vi "Wertaenderung Systemeinstellungen.vi"(11 "error in (no error)":errorcluster caption="Fehler (Eingang, kein Fehler)", 13 "Aktion":T1) -> (4 "Tests":T2, 15 "error out":errorcluster caption="Fehler (Ausgang)")   [LabVIEW 2020, in "EPA 1065.lvlib"]
uses:
  EPA 1065.lvlib
  Aktive Tests Cluster.ctl
  Aktion Wertaenderung Gasliste.ctl
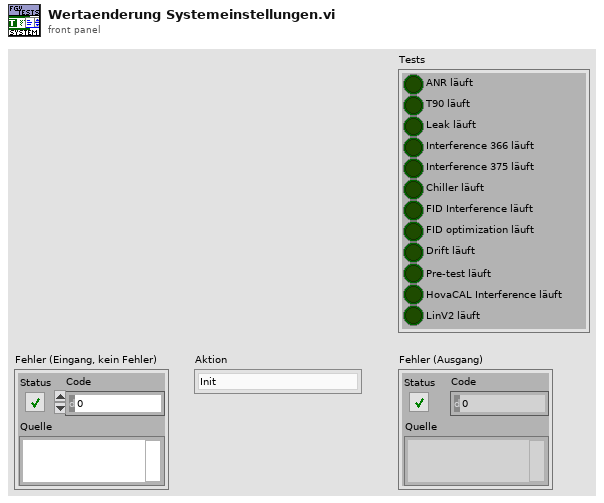
[diagram p1: front panel]
types:
  T1 = typedef "EPA 1065.lvlib/Aktion Wertaenderung Gasliste.ctl" = enum16{"Init", "lesen", "Gasliste geändert", "ARN inaktiv", "LEAK inaktiv", "Interference 366 inaktiv", "T90 inaktiv", "Interference 375 inaktiv", "Chiller inaktiv", "FID O2 inaktiv", "FID Opti inaktiv", "Drift inaktiv", "Pre Test inaktiv", "LinV2 inaktiv", "HovaCAL Interference inaktiv"}
  T2 = typedef "EPA 1065.lvlib/Aktive Tests Cluster.ctl" = cluster{"ANR läuft":bool, "T90 läuft":bool, "Leak läuft":bool, "Interference 366 läuft":bool, "Interference 375 läuft":bool, "Chiller läuft":bool, "FID Interference läuft":bool, "FID optimization läuft":bool, "Drift läuft":bool, "Pre-test läuft":bool, "HovaCAL Interference läuft":bool, "LinV2 läuft":bool}
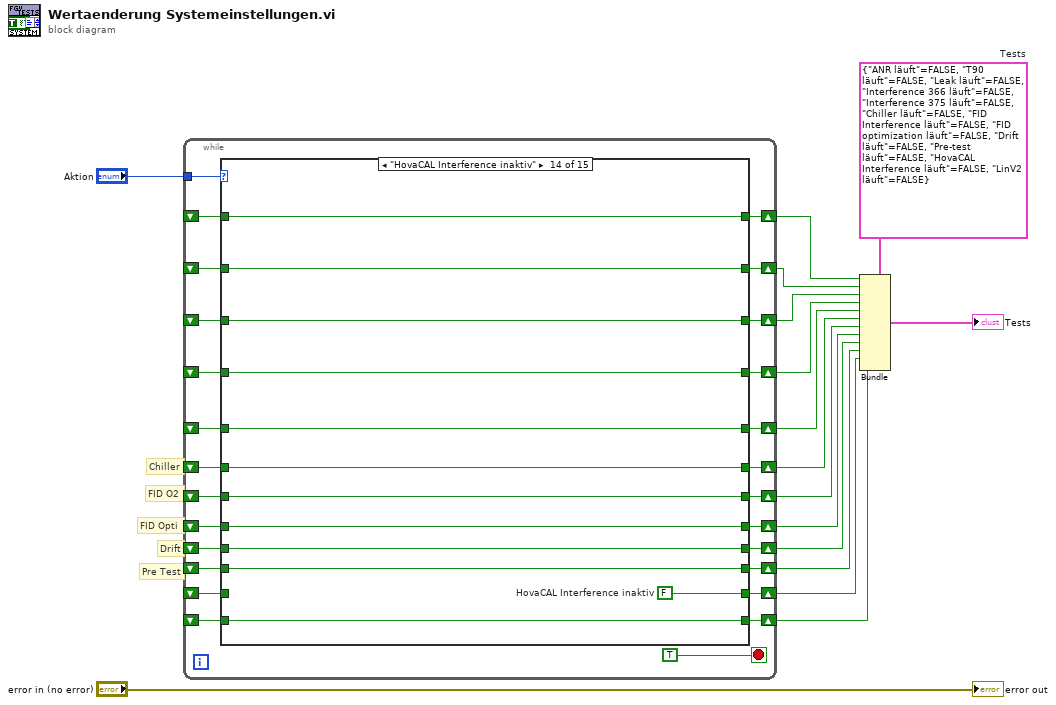
[diagram p0: block diagram]
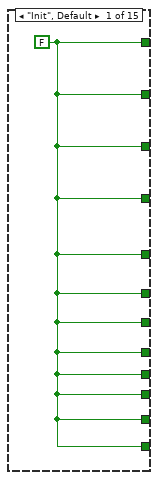
[diagram p2: hidden frame]
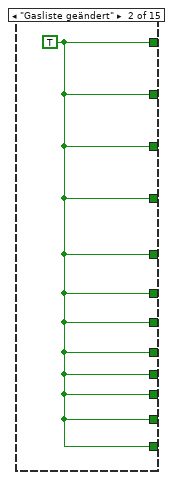
[diagram p3: hidden frame]
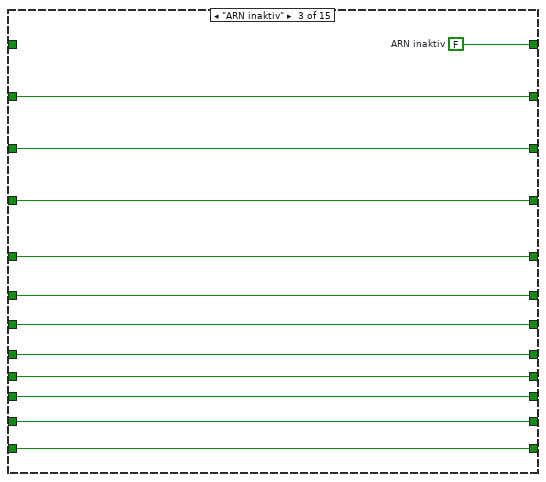
[diagram p4: hidden frame]
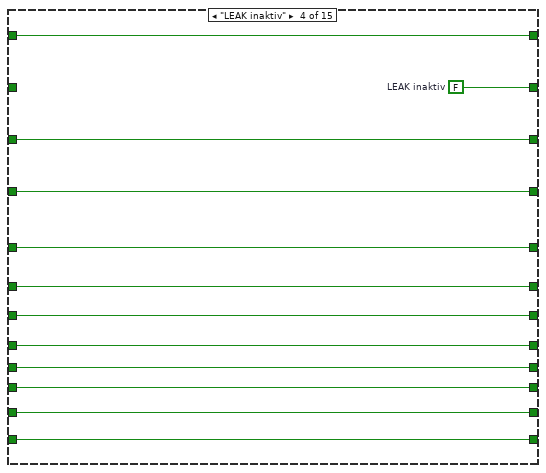
[diagram p5: hidden frame]
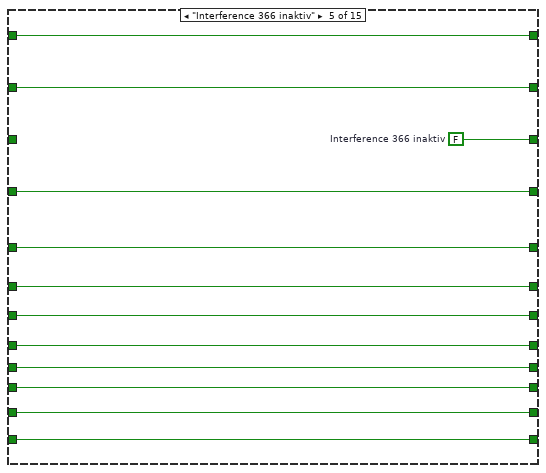
[diagram p6: hidden frame]
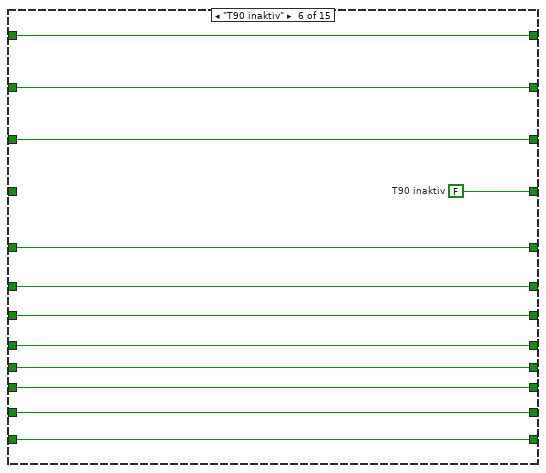
[diagram p7: hidden frame]
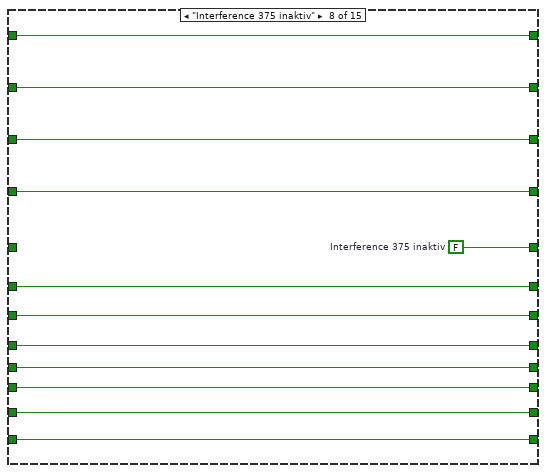
[diagram p9: hidden frame]
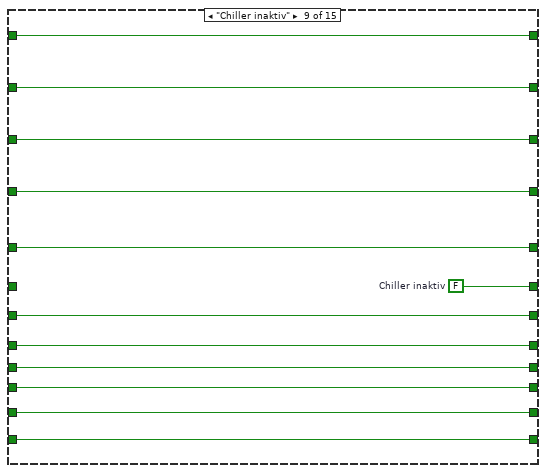
[diagram p10: hidden frame]
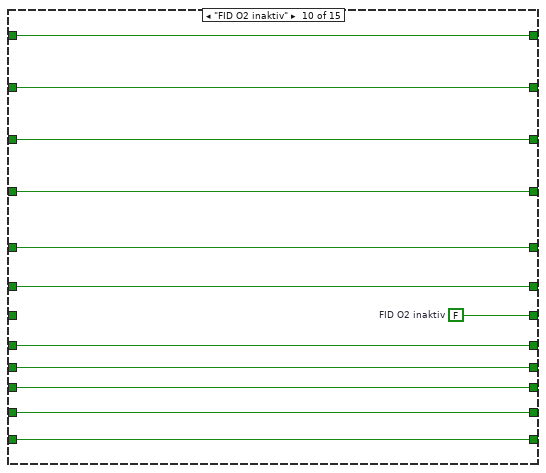
[diagram p11: hidden frame]
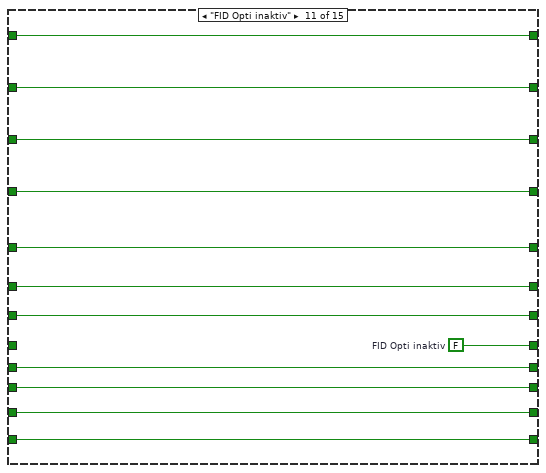
[diagram p12: hidden frame]
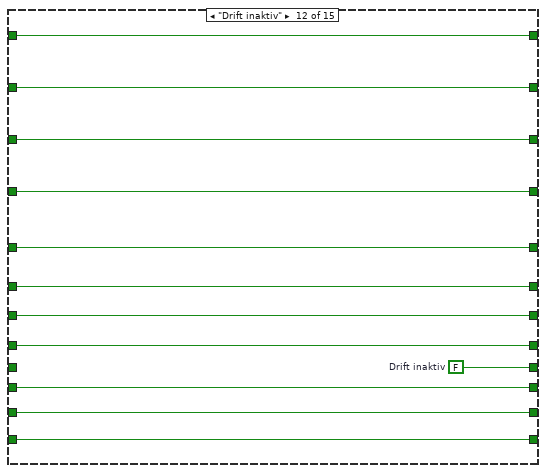
[diagram p13: hidden frame]
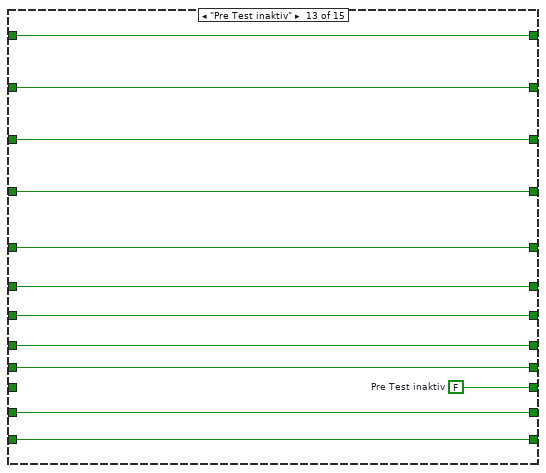
[diagram p14: hidden frame]
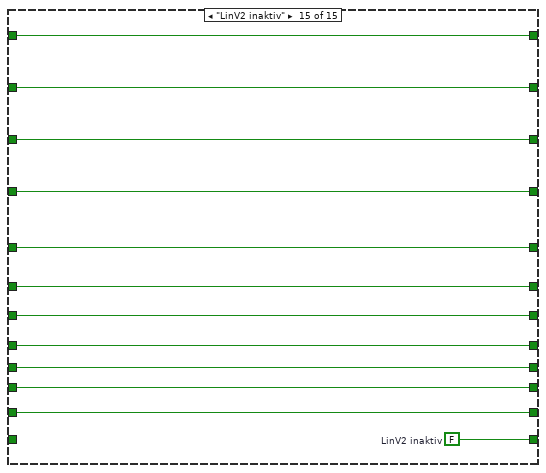
[diagram p15: hidden frame]
diagram:
  w4 = T2 {"ANR läuft"=FALSE, "T90 läuft"=FALSE, "Leak läuft"=FALSE, "Interference 366 läuft"=FALSE, "Interference 375 läuft"=FALSE, "Chiller läuft"=FALSE, "FID Interference läuft"=FALSE, "FID optimization läuft"=FALSE, "Drift läuft"=FALSE, "Pre-test läuft"=FALSE, "HovaCAL Interference läuft"=FALSE, "LinV2 läuft"=FALSE}  # Tests
  # "Pre Test"
  # "Drift"
  # "FID Opti"
  # "FID O2"
  # "Chiller"
  n1 = while {
    tunnel: "Aktion" -> [w41]
    shift-right: [w40] -> w7
    shift-left: _ -> [w36]
    shift-right: [w39] -> w8
    shift-left: _ -> [w35]
    shift-right: [w38] -> w9
    shift-left: _ -> [w34]
    shift-right: [w37] -> w10
    shift-left: _ -> [w33]
    shift-right: [w31] -> w11
    shift-left: _ -> [w32]
    shift-right: [w30] -> w12
    shift-left: _ -> [w29]
    shift-right: [w27] -> w13
    shift-left: _ -> [w28]
    shift-right: [w26] -> w14
    shift-left: _ -> [w25]
    shift-right: [w23] -> w15
    shift-left: _ -> [w24]
    shift-right: [w22] -> w16
    shift-left: _ -> [w21]
    shift-right: [w20] -> w2
    shift-left: _ -> [w19]
    shift-right: [w18] -> w1
    shift-left: _ -> [w17]
    stop <- TRUE stop-if-true
    n2 = case shown="\"HovaCAL Interference inaktiv\"" w41 {
      tunnel: [w43 w44 w56 w67 w80 w92 w104 w116 w128 w140 w152 w164 w176 w188 w200] -> w40
      tunnel: [w43 w44 w55 w68 w79 w91 w103 w115 w127 w139 w151 w163 w175 w187 w199] -> w39
      tunnel: [w43 w44 w54 w66 w78 w90 w102 w114 w126 w138 w150 w162 w174 w186 w198] -> w38
      tunnel: [w43 w44 w53 w65 w77 w89 w101 w113 w125 w137 w149 w161 w173 w185 w197] -> w37
      tunnel: w36 -> [_ _ _ w67 w80 w92 w104 w116 w128 w140 w152 w164 w176 w188 w200]
      tunnel: w35 -> [_ _ w55 _ w79 w91 w103 w115 w127 w139 w151 w163 w175 w187 w199]
      tunnel: w34 -> [_ _ w54 w66 _ w90 w102 w114 w126 w138 w150 w162 w174 w186 w198]
      tunnel: w33 -> [_ _ w53 w65 w77 _ w101 w113 w125 w137 w149 w161 w173 w185 w197]
      tunnel: [w43 w44 w52 w64 w76 w88 w100 w112 w124 w136 w148 w160 w172 w184 w196] -> w31
      tunnel: w32 -> [_ _ w52 w64 w76 w88 w100 _ w124 w136 w148 w160 w172 w184 w196]
      tunnel: [w43 w44 w51 w63 w75 w87 w99 w111 w119 w135 w147 w159 w171 w183 w195] -> w30
      tunnel: w29 -> [_ _ w51 w63 w75 w87 w99 w111 _ w135 w147 w159 w171 w183 w195]
      tunnel: [w43 w44 w50 w62 w74 w86 w98 w110 w123 w131 w146 w158 w170 w182 w194] -> w27
      tunnel: w28 -> [_ _ w50 w62 w74 w86 w98 w110 w123 _ w146 w158 w170 w182 w194]
      tunnel: [w43 w44 w49 w61 w73 w85 w97 w109 w122 w134 w143 w157 w169 w181 w193] -> w26
      tunnel: w25 -> [_ _ w49 w61 w73 w85 w97 w109 w122 w134 _ w157 w169 w181 w193]
      tunnel: [w43 w44 w48 w60 w72 w84 w96 w108 w121 w133 w145 w156 w168 w180 w192] -> w23
      tunnel: w24 -> [_ _ w48 w60 w72 w84 w96 w108 w121 w133 w145 _ w168 w180 w192]
      tunnel: [w43 w44 w47 w59 w71 w83 w95 w107 w120 w132 w144 w155 w167 w179 w191] -> w22
      tunnel: w21 -> [_ _ w47 w59 w71 w83 w95 w107 w120 w132 w144 w155 _ w179 w191]
      tunnel: [w43 w44 w46 w58 w70 w82 w94 w106 w118 w130 w142 w154 w166 w177 w190] -> w20
      tunnel: w19 -> [_ _ w46 w58 w70 w82 w94 w106 w118 w130 w142 w154 w166 w177 _]
      tunnel: [w43 w44 w45 w57 w69 w81 w93 w105 w117 w129 w141 w153 w165 w178 w189] -> w18
      tunnel: w17 -> [_ _ w45 w57 w69 w81 w93 w105 w117 w129 w141 w153 w165 _ w189]
      frame "Init", Default {
        w43 = FALSE
      }
      frame "Gasliste geändert" {
        w44 = TRUE
      }
      frame "ARN inaktiv" {
        w56 = FALSE  # ARN inaktiv
      }
      frame "LEAK inaktiv" {
        w68 = FALSE  # LEAK inaktiv
      }
      frame "Interference 366 inaktiv" {
        w78 = FALSE  # Interference 366 inaktiv
      }
      frame "T90 inaktiv" {
        w89 = FALSE  # T90 inaktiv
      }
      frame "lesen" {
      }
      frame "Interference 375 inaktiv" {
        w112 = FALSE  # Interference 375 inaktiv
      }
      frame "Chiller inaktiv" {
        w119 = FALSE  # Chiller inaktiv
      }
      frame "FID O2 inaktiv" {
        w131 = FALSE  # FID O2 inaktiv
      }
      frame "FID Opti inaktiv" {
        w143 = FALSE  # FID Opti inaktiv
      }
      frame "Drift inaktiv" {
        w156 = FALSE  # Drift inaktiv
      }
      frame "Pre Test inaktiv" {
        w167 = FALSE  # Pre Test inaktiv
      }
      frame "HovaCAL Interference inaktiv" {
        w178 = FALSE  # HovaCAL Interference inaktiv
      }
      frame "LinV2 inaktiv" {
        w190 = FALSE  # LinV2 inaktiv
      }
    }
  }
  n3 = Bundle(cluster=w4, "ANR läuft"=w7, "T90 läuft"=w8, "Leak läuft"=w9, "Interference 366 läuft"=w10, "Interference 375 läuft"=w11, "Chiller läuft"=w12, "FID Interference läuft"=w13, "FID optimization läuft"=w14, "Drift läuft"=w15, "Pre-test läuft"=w16, "HovaCAL Interference läuft"=w1, "LinV2 läuft"=w2) -> (→"Tests":T2)
  "error out" <- "error in (no error)"
